vi "test_serialize_deserialize.vi"   [LabVIEW 2020, in "NI_ADAS_CAN.lvlib"]
doc: "Version 0.1"
uses:
  NI_ADAS_CAN.lvlib
  <vilib>/addons/_JKI Toolkits/Caraya/classes/Test/Test.lvclass
  <vilib>/addons/_JKI Toolkits/Caraya/classes/Assert/Assert.lvclass
  Serialize Data.vi
  Process Data.ctl
  <vilib>/xnet/xnet.llb/XNET Frame Type CAN.ctl
  <vilib>/xnet/xnet.llb/XNET Frame CAN.ctl
  ADAS Generic/Deserialize Data.vi
  ADAS Generic/NI_ADAS_Generic.lvlib
types:
  T1 = typedef "NI_ADAS_CAN.lvlib/Process Data.ctl" = cluster{"Timestamp":timestamp, "Bus Channel":u16, "CAN Frame Array":T2[]}
  T2 = typedef "XNET Frame CAN.ctl" = cluster{"timestamp":timestamp, "payload":u8[], "identifier":u32, "type":T3, "extended?":bool, "echo?":bool}
  T3 = typedef "XNET Frame Type CAN.ctl" = u8
  T4 = typedef "NI_ADAS_Generic.lvlib/Process Data.ctl" = cluster{"Timestamp":timestamp, "Bus Channel":u16, "Byte Array":u8[]}
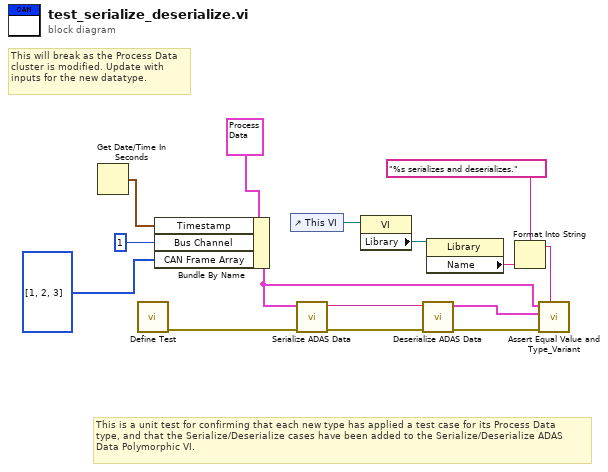
[diagram p0: block diagram]
diagram:
  # "This will break as the Process Data\ncluster is modified. Update with\ninputs for the new datatype."
  # "This is a unit test for confirming that each new type has applied a test case for its Process Data\ntype, and that the Serialize/Deserialize cases have been added to the Serialize/Deserialize ADAS\nData Polymorphic VI."
  n1 = Get Date/Time In Seconds() -> (seconds since 1Jan1904=w4:timestamp)
  n2 = call <vilib>:"Define Test.vi"() -> ("error out"=w10:errorcluster)  [unwired: 11 in]
  n3 = Bundle By Name(cluster=T1 {"Timestamp"=timestamp(0 s since 1904-01-01), "Bus Channel"=0, "CAN Frame Array"=[]} ("Process Data in"), "Timestamp"=w4, "Bus Channel"=u16 1, "CAN Frame Array"=u8[] [1, 2, 3] ("Byte Array")) -> (w1:T1)
  n4 = control-ref of="This VI"() -> (w15:refnum<vi>)
  n5 = call-poly "Serialize ADAS Data.vi"("error in (no error)"=w10, "Process Data"=w1) -> ("error out"=w9:errorcluster, "Flat Data out"=w8:string)  [unwired: 8 in]
  n6 = property class="VI"(reference=w15) -> ("Library"=w14:refnum<vi>)  [unwired: 1 in, 2 out]
  n7 = call-poly "Deserialize ADAS Data.vi"("error in (no error)"=w9, "Flat Data in"=w8) -> ("error out"=w6:errorcluster, "Process Data out"=w7:T4)  [unwired: 8 in]
  n8 = property class="Library"(reference=w14) -> ("Name"=w12:string)  [unwired: 1 in, 2 out]
  n9 = Format Into String(format string="%s serializes and deserializes.", w12) -> (resulting string=w11:string)  [unwired: 2 in, 1 out]
  n10 = call <vilib>:"Assert Equal Value and Type_Variant.vi"("Label"=w11, "error in (no error)"=w6, "Y"=w7, "X"=w1) -> ()  [unwired: 7 in, 1 out]
